vi "StandardMHL.vi"(8 "error in (no error)":errorcluster, 9 "Message Data":variant, 10 "Message":string, 11 "JQMHModule in":refnum<class "JQMHModule.lvclass">) -> (0 "error out":errorcluster, 3 "JQMHModule out":refnum<class "JQMHModule.lvclass">)   [LabVIEW 2024, in "JQMHModule.lvclass"]
uses:
  JQMHModule.lvclass
  JQMHModule.lvclass/JQMHModule.ctl
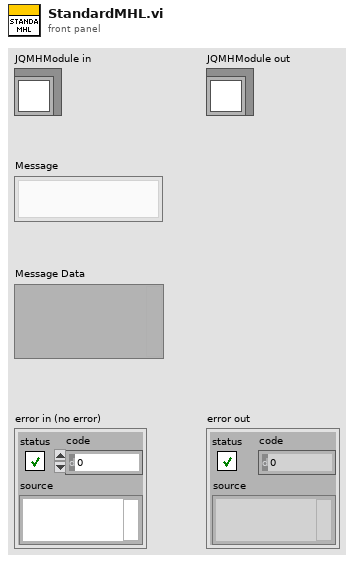
[diagram p1: front panel]
types:
  T1 = typedef "JQMHModule.lvclass/StandardEvents.ctl" = cluster{"Stop Module":refnum<user-event>}
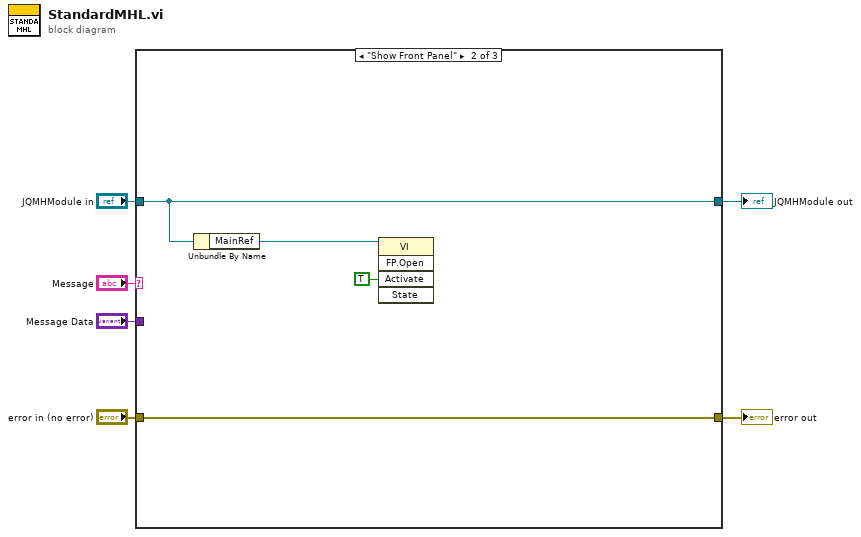
[diagram p0: block diagram]
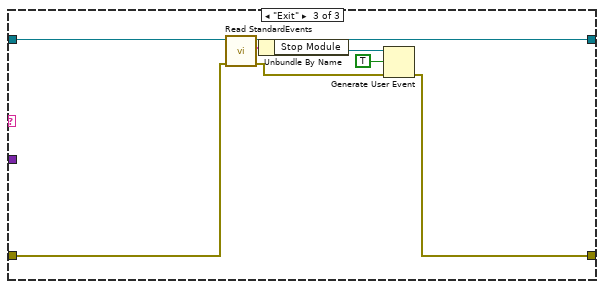
[diagram p3: hidden frame]
diagram:
  n1 = case shown="\"Show Front Panel\"" "Message" {
    tunnel: "Message Data" -> [_ _ _]
    tunnel: "JQMHModule in" -> [w8 w11 w16]
    tunnel: "error in (no error)" -> [w7 w12 w15]
    tunnel: [w7 w12 w14] -> w2
    tunnel: [w8 w11 w13] -> w1
    frame Default {
    }
    frame "Show Front Panel" {
      n2 = Unbundle By Name(w11) -> ("MainRef"=w10:refnum<vi>)
      n3 = invoke class="VI" method="FP.Open"(reference=w10, "Activate"=TRUE ("Activate?")) -> ()  [unwired: 3 in, 5 out]
    }
    frame "Exit" {
      n4 = call "Read StandardEvents.vi"("error in (no error)"=w15, "JQMHCore in"=w16) -> ("error out"=w17:errorcluster, "StandardEvents"=w20:T1, "JQMHCore out"=w13:refnum<class "JQMHModule.lvclass">)  [unwired: 7 in]
      n5 = Unbundle By Name(w20) -> ("Stop Module"=w19:refnum<user-event>)
      n6 = Generate User Event(user event=w19, event data cluster=TRUE, error in=w17) -> (error out=w14:errorcluster)  [unwired: 1 in, 1 out]
    }
  }
  "error out" <- w2
  "JQMHModule out" <- w1
